vi "DAQ.Calibrate.vi"(8 "error in (no error)":errorcluster, 11 "Lockin.DAQ in":refnum<class "Instrument.DAQ.lvclass">) -> (0 "error out":errorcluster, 2 "Cal Info":T1[](array[typedef]) {"DevTemp" format="%.1f"; "SelfCal.LastTemp" format="%.1f"; "SelfCal.LastDate/Time" format="%<%I:%M %p %m/%d/%Y>T"}, 3 "Lockin.DAQ out":refnum<class "Instrument.DAQ.lvclass">)   [LabVIEW 2019, in "Instrument.Lockin.lvlib" / "Instrument.DAQ.lvclass"]
uses:
  Instrument.DAQ.lvclass
  Typedefs/DAQ.Calibration--Cluster.ctl
  <vilib>/addons/WireFlow/_WF_ProgressBar.llb/WindowBehavior.ctl
  Instrument.DAQ.lvclass/Instrument.DAQ.ctl
  <vilib>/addons/WireFlow/_WF_ProgressBar.llb/ProgressBar_WireFlow.lvclass
  <resource>/objmgr/daqmx.rc
panel:
  out "Numeric":i32
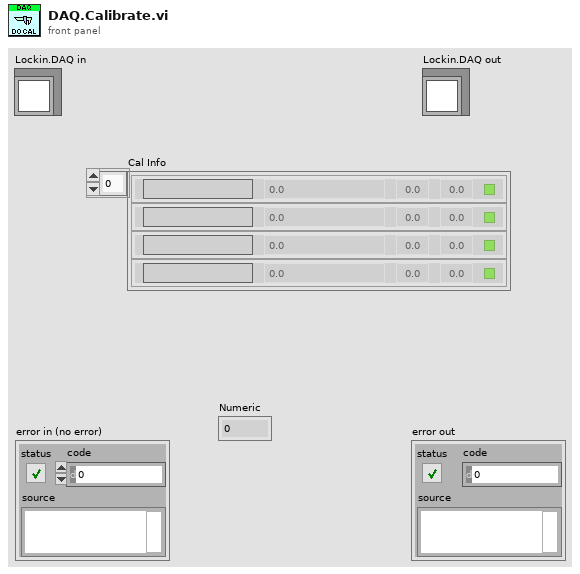
[diagram p1: front panel]
types:
  T1 = typedef "Instrument.Lockin.lvlib/Instrument.DAQ.lvclass/DAQ.Calibration--Cluster.ctl" = cluster{"Active Device":string, "SelfCal.LastDate/Time":dbl, "SelfCal.LastTemp":dbl, "DevTemp":dbl, "calibration due?":bool}
  T2 = typedef "ProgressBar_WireFlow.lvclass/WindowBehavior.ctl" = enum16{"No change", "Modal", "Floating"}
  T3 = typedef "Instrument.Lockin.lvlib/Instrument.DAQ.lvclass/DAQ.Calibration--Cluster--Array.ctl" = T1[]
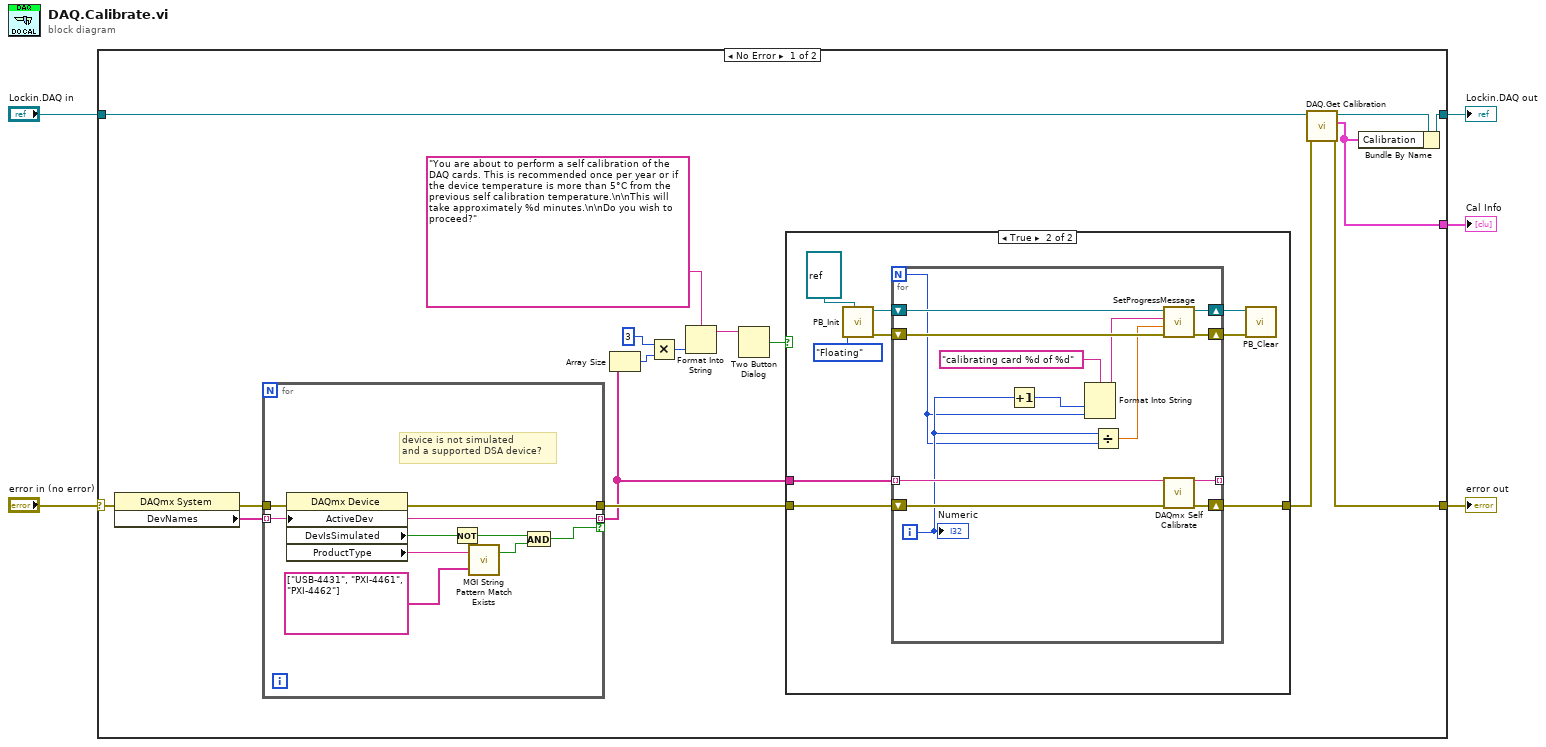
[diagram p0: block diagram]
diagram:
  n1 = case shown="No Error" "error in (no error)" {
    selector: "error in (no error)" -> [w7 w56]
    tunnel: [w22 w55] -> w5
    tunnel: [w19 w56] -> w4
    tunnel: "Lockin.DAQ in" -> [w17 w55]
    tunnel: [w6 _] -> w2
    frame No Error {
      n2 = property class="DAQmx System"(error in=w7) -> (error out=w14:errorcluster, "DevNames"=w15:tag[])  [unwired: 1 in, 1 out]
      n3 = for {
        tunnel: [w26] -> w10 mode=indexing if=w24
        tunnel: w15 -> [w26] mode=indexing
        tunnel: w14 -> [w25]
        tunnel: [w23] -> w13
        # "device is not simulated\nand a supported DSA device?"
        n4 = property class="DAQmx Device"(error in=w25, "ActiveDev"=w26) -> (error out=w23:errorcluster, "DevIsSimulated"=w31:bool, "ProductType"=w28:string)  [unwired: 1 in, 1 out]
        n5 = Not(x=w31) -> (.not. x?=w30:bool)
        n6 = call <userlib>:"MGI String Pattern Match Exists.vi"("Patterns to Try"=string[] ["USB-4431", "PXI-4461", "PXI-4462"], "String"=w28) -> ("Match Found"=w27:bool)  [unwired: 1 out]
        n7 = And(x=w30, y=w27) -> (x .and. y?=w24:bool)
      }
      n8 = Array Size(array=w10) -> (size(s)=w12:i32)
      n9 = Multiply(x=3, y=w12) -> (x*y=w9:i32)
      n10 = Format Into String(format string="You are about to perform a self calibration of the DAQ cards. This is recommended once per year or if the device temperature is more than 5°C from the previous self calibration temperature.\n\nThis will take approximately %d minutes.\n\nDo you wish to proceed?" ("message"), w9) -> (resulting string=w8:string)  [unwired: 2 in, 1 out]
      n11 = Two Button Dialog(message=w8) -> (T button?=w20:bool)  [unwired: 2 in]
      n12 = case shown="True" w20 {
        tunnel: w13 -> [w32 w41]
        tunnel: [w32 w40] -> w18
        tunnel: w10 -> [_ w39]
        frame False {
        }
        frame True {
          n13 = call <vilib>:"PB_Init.vi"("Progress VI"=refnum<vi> refnum, "Window behavior (No change)"=WindowBehavior."Floating") -> ("error out"=w35:errorcluster, "WF-ProgressBar out"=w36:refnum<class "ProgressBar_WireFlow.lvclass">)  [unwired: 8 in]
          n14 = for {
            N -> [w44]
            shift-right: [w53] -> w40
            shift-left: w41 -> [w54]
            tunnel: w39 -> [w52] mode=indexing
            tunnel: [w52] -> _ mode=indexing
            shift-right: [w49] -> w38
            shift-left: w36 -> [w50]
            shift-right: [w48] -> w37
            shift-left: w35 -> [w51]
            i -> [w46]
            n15 = Increment(x=w46) -> (x+1=w43:i32)
            n16 = Format Into String(format string="calibrating card %d of %d", w43, w44) -> (resulting string=w42:string)  [unwired: 2 in, 1 out]
            n17 = Divide(x=w46, y=w44) -> (x/y=w47:dbl)
            n18 = call-dynamic "SetProgressMessage.vi"("error in (no error)"=w51, "Progress value (NaN no update)"=w47, "Message"=w42, "WF-ProgressBar in"=w50) -> ("error out"=w48:errorcluster, "WF-ProgressBar out"=w49:refnum<class "ProgressBar_WireFlow.lvclass">)  [unwired: 5 in, 1 out]
            n19 = call <vilib>:"DAQmx Self Calibrate.vi"("device in"=w52, "error in"=w54) -> ("error out"=w53:errorcluster)  [unwired: 13 in]
            "Numeric" <- w46
          }
          n20 = call-dynamic "PB_Clear.vi"("error in (no error)"=w37, "WF-ProgressBar in"=w38) -> ()  [unwired: 8 in, 2 out]
        }
      }
      n21 = call "DAQ.Get Calibration.vi"("error in (no error)"=w18, "Instrument.DAQ in"=w17) -> ("error out"=w19:errorcluster, "Calibration"=w6:T3, "Instrument.DAQ out"=w16:refnum<class "Instrument.DAQ.lvclass">)  [unwired: 7 in]
      n22 = Bundle By Name(cluster=w16, "Calibration"=w6) -> (w22:refnum<class "Instrument.DAQ.lvclass">)
    }
    frame Error {
    }
  }
  "error out" <- w4
  "Cal Info" <- w2
  "Lockin.DAQ out" <- w5
